vi "FRCts20_WebMethods_Convert_Team.vi"(8 "error in (no error)":errorcluster, 11 "Team Out":T1) -> (0 "error out":errorcluster, 3 "Team":T4)   [LabVIEW 2014, in "FRCts20_WebMethods.lvlib"]
uses:
  FRCts20_WebMethods.lvlib
  ESP Engine/source/VI Source/TypeDefs/FRCts20_EspEngine_Team.ctl
  Web Method Public Interface/FRCts20_WebMethods_ctl_singleTeam.ctl
  Web Method Public Interface/FRCts20_WebMethods_ctl_teamIdentifier.ctl
  Backend/source/VI Source/FRCts20_Backend_API/FRCts20_Backend_API_SW.ctl
  Web Method Public Interface/FRCts20_WebMethods_ctl_request.ctl
  Backend/source/VI Source/FRCts20_Backend_API/FRCts20_Backend_API_Status.ctl
  Backend/source/VI Source/FRCts20_Backend_API/FRCts20_Backend_API_Team.ctl
  Backend/source/VI Source/FRCts20_Backend_API/FRCts20_Backend_API.lvlib
  ESP Engine/source/VI Source/FRCts20_EspEngine.lvlib
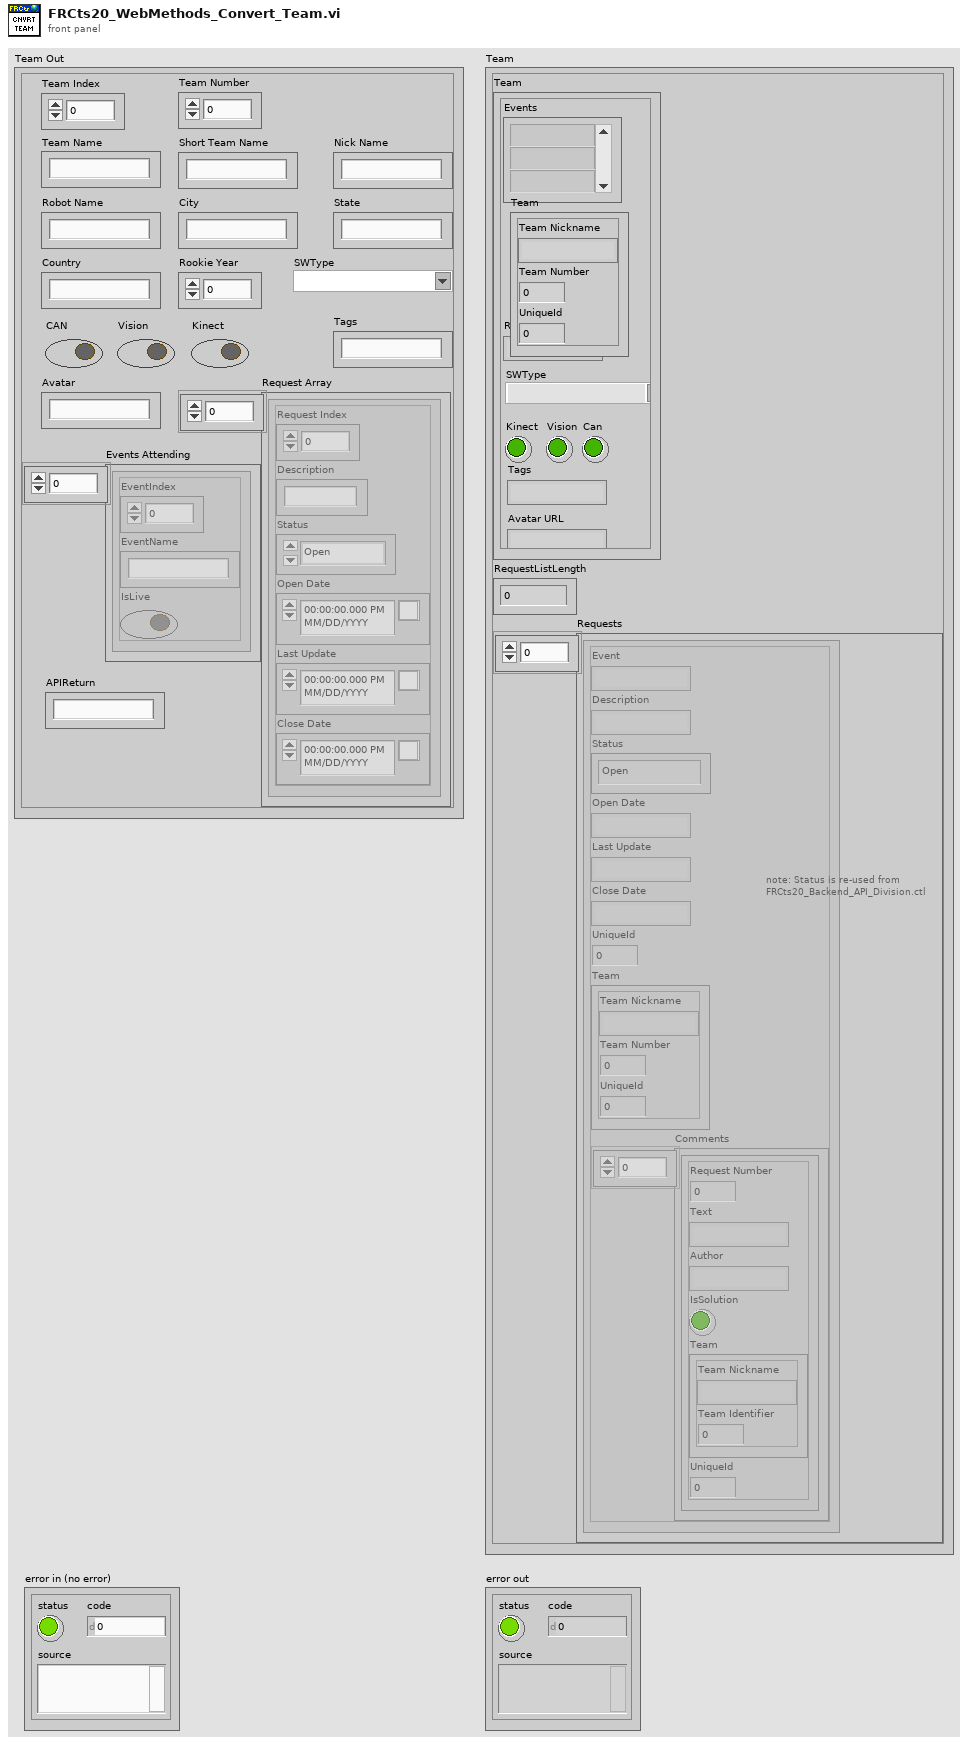
[diagram p1: front panel]
types:
  T1 = typedef "FRCts20_Backend_API.lvlib/FRCts20_Backend_API_Team.ctl" = cluster{"Team Index":u32, "Team Number":u32, "Team Name":string, "Short Team Name":string, "Nick Name":string, "Robot Name":string, "City":string, "State":string, "Country":string, "Rookie Year":u32, "SWType":T2, "CAN":bool, "Vision":bool, "Kinect":bool, "Tags":string, "Avatar":string, "Request Array":cluster{"Request Index":u32, "Description":string, "Status":T3, "Open Date":timestamp, "Last Update":timestamp, "Close Date":timestamp}[], "Events Attending":cluster{"EventIndex":dbl, "EventName":string, "IsLive":bool}[], "APIReturn":string}
  T2 = typedef "FRCts20_Backend_API.lvlib/FRCts20_Backend_API_SW.ctl" = string
  T3 = typedef "FRCts20_Backend_API.lvlib/FRCts20_Backend_API_Status.ctl" = enum16{"Open", "In Work", "Closed"}
  T4 = typedef "FRCts20_EspEngine.lvlib/FRCts20_EspEngine_Team.ctl" = cluster{"Team":T5, "RequestListLength":i16, "Requests":T7[]}
  T5 = typedef "FRCts20_WebMethods.lvlib/FRCts20_WebMethods_ctl_singleTeam.ctl" = cluster{"Events":string[], "Robot Name":string, "Kinect":bool, "Vision":bool, "Can":bool, "Tags":string, "Avatar URL":string, "Team":T6, "SWType":T2}
  T6 = typedef "FRCts20_WebMethods.lvlib/FRCts20_WebMethods_ctl_teamIdentifier.ctl" = cluster{"Team Nickname":string, "Team Number ":u32, "UniqueId":u32}
  T7 = typedef "FRCts20_WebMethods.lvlib/FRCts20_WebMethods_ctl_request.ctl" = cluster{"Event":string, "Description":string, "Status":T3, "Open Date":string, "Last Update":string, "Close Date":string, "UniqueId":i32, "Team":cluster{"Team Nickname":string, "Team Number ":i32, "UniqueId":i32}, "Comments":cluster{"Request Number":dbl, "Text":string, "Author":string, "IsSolution":bool, "Team":cluster{"Team Nickname":string, "Team Identifier ":dbl}, "UniqueId":i32}[]}
  T8 = cluster{"Request Index":u32, "Description":string, "Status":T3, "Open Date":timestamp, "Last Update":timestamp, "Close Date":timestamp}[]
  T9 = cluster{"EventIndex":dbl, "EventName":string, "IsLive":bool}[]
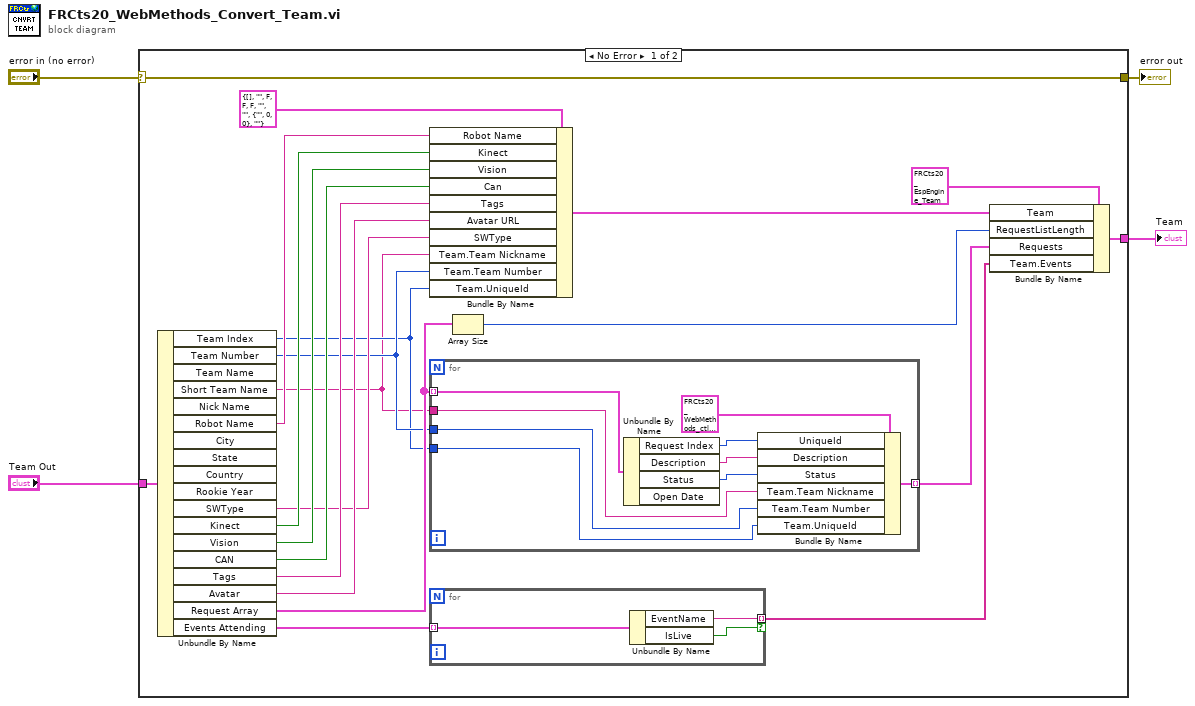
[diagram p0: block diagram]
diagram:
  n1 = case shown="No Error" "error in (no error)" {
    selector: "error in (no error)" -> [w8 w38]
    tunnel: [w8 w38] -> w1
    tunnel: "Team Out" -> [w10 _]
    tunnel: [w9 _] -> w3
    frame No Error {
      n2 = Unbundle By Name(w10) -> ("Team Index"=w12:u32, "Team Number"=w13:u32, "Short Team Name"=w7:string, "Robot Name"=w21:string, "SWType"=w15:T2, "Kinect"=w20:bool, "Vision"=w19:bool, "CAN"=w18:bool, "Tags"=w17:string, "Avatar"=w16:string, "Request Array"=w14:T8, "Events Attending"=w6:T9)  [unwired: 6 out]
      n3 = Bundle By Name(cluster=T5 {"Events"=[], "Robot Name"="", "Kinect"=FALSE, "Vision"=FALSE, "Can"=FALSE, "Tags"="", "Avatar URL"="", "Team"={"Team Nickname"="", "Team Number "=0, "UniqueId"=0}, "SWType"=""} ("Team"), "Robot Name"=w21, "Kinect"=w20, "Vision"=w19, "Can"=w18, "Tags"=w17, "Avatar URL"=w16, "SWType"=w15, "Team.Team Nickname"=w7, "Team.Team Number"=w13, "Team.UniqueId"=w12) -> (w22:T5)
      n4 = for {
        tunnel: w14 -> [w37] mode=indexing
        tunnel: w7 -> [w32]
        tunnel: w13 -> [w31]
        tunnel: w12 -> [w30]
        tunnel: [w29] -> w11 mode=indexing
        n5 = Unbundle By Name(w37) -> ("Request Index"=w35:u32, "Description"=w34:string, "Status"=w33:T3)  [unwired: 1 out]
        n6 = Bundle By Name(cluster=T7 {"Event"="", "Description"="", "Status"=enum."Open", "Open Date"="", "Last Update"="", "Close Date"="", "UniqueId"=0, "Team"={"Team Nickname"="", "Team Number "=0, "UniqueId"=0}, "Comments"=[]} ("Request"), "UniqueId"=w35, "Description"=w34, "Status"=w33, "Team.Team Nickname"=w32, "Team.Team Number"=w31, "Team.UniqueId"=w30) -> (w29:T7)
      }
      n7 = for {
        tunnel: w6 -> [w28] mode=indexing
        tunnel: [w27] -> w5 mode=indexing if=w26
        n8 = Unbundle By Name(w28) -> ("EventName"=w27:string, "IsLive"=w26:bool)
      }
      n9 = Array Size(array=w14) -> (size(s)=w24:i32)
      n10 = Bundle By Name(cluster=T4 {"Team"={"Events"=[], "Robot Name"="", "Kinect"=FALSE, "Vision"=FALSE, "Can"=FALSE, "Tags"="", "Avatar URL"="", "Team"={"Team Nickname"="", "Team Number "=0, "UniqueId"=0}, "SWType"=""}, "RequestListLength"=0, "Requests"=[]} ("Team"), "Team"=w22, "RequestListLength"=w24, "Requests"=w11, "Team.Events"=w5) -> (w9:T4)
    }
    frame Error {
    }
  }
  "Team" <- w3
  "error out" <- w1
